vi "advent_5.vi"() -> ()   [LabVIEW 2021]
uses:
  <vilib>/Utility/file.llb/Read Delimited Spreadsheet (string).vi
panel:
  out "answer":i32
  out "Array 2":i32[][](array[numeric])
  out "Array":i32[][](array[numeric])
  out "ey":string[](array[string])
  out "ex":string[](array[string])
  out "e":string[](array[string])
  out "s":string[](array[string])
  out "sy":string[](array[string])
  out "sx":string[](array[string])
  out "all rows":string[][](array[string])
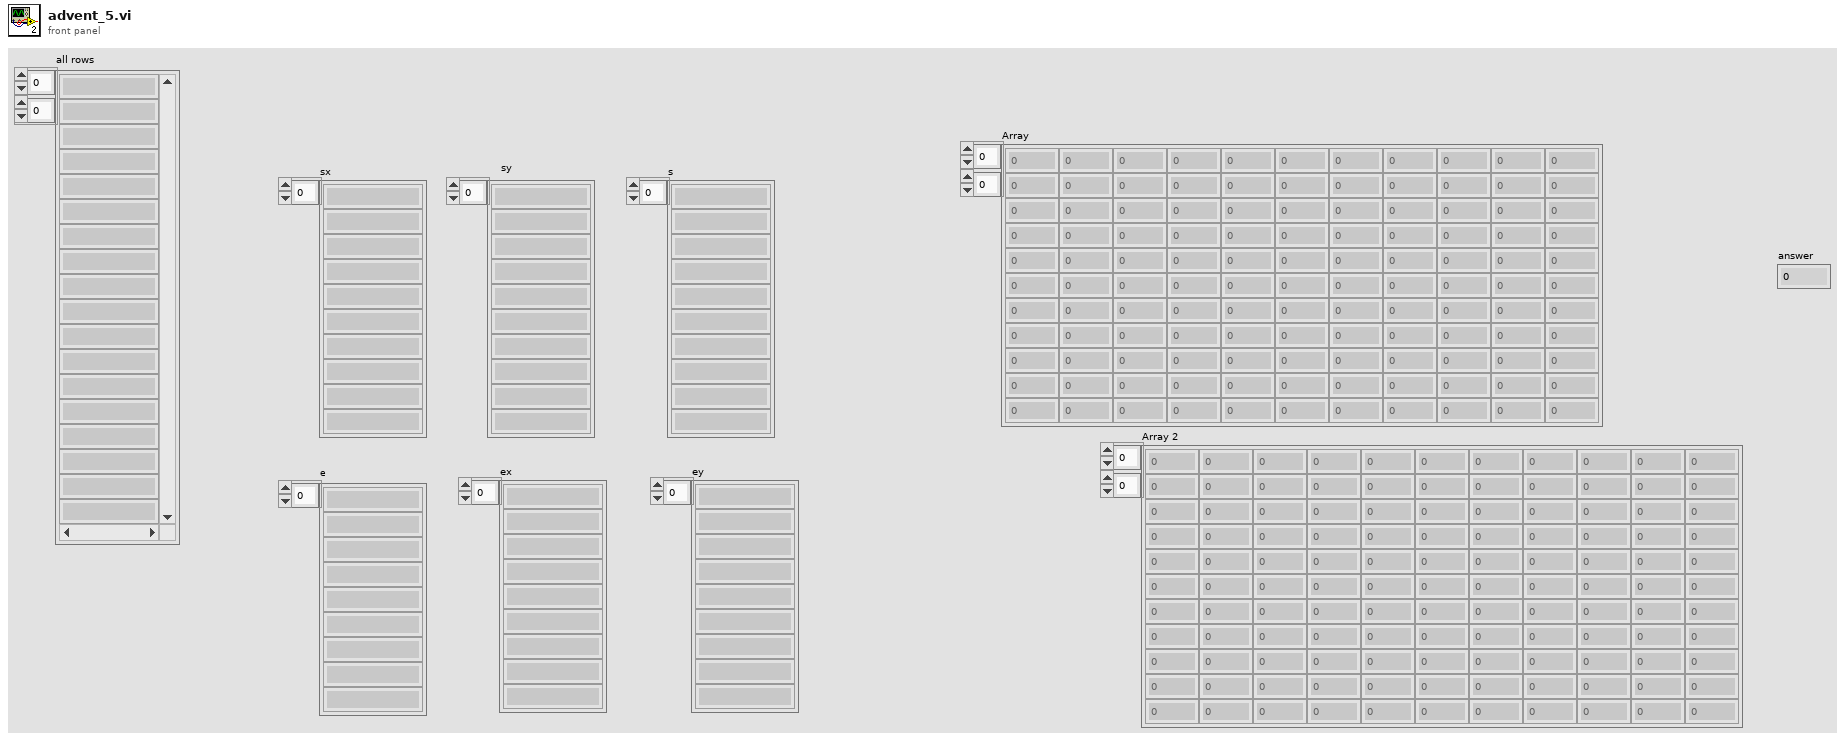
[diagram p1: front panel]
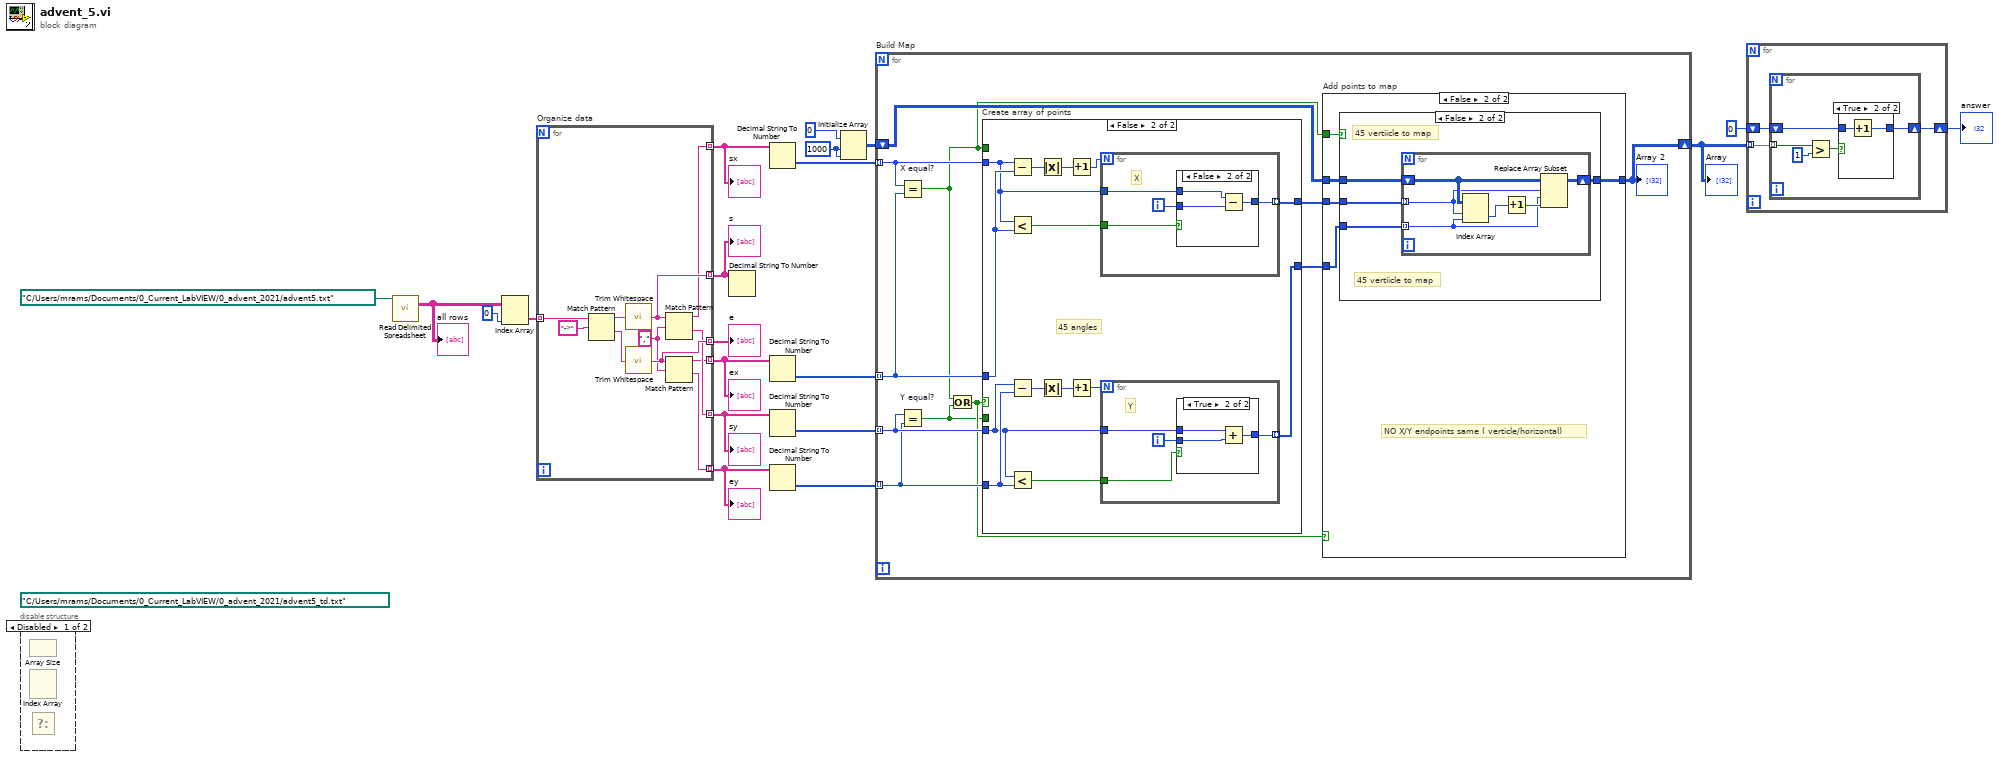
[diagram p0: block diagram]
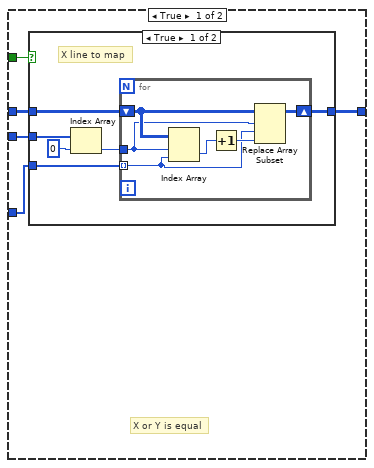
[diagram p3: hidden frame]
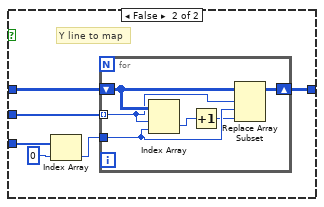
[diagram p4: hidden frame]
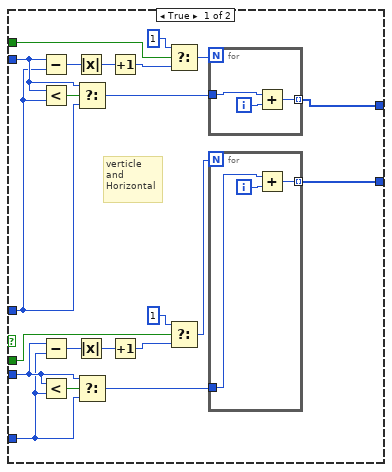
[diagram p6: hidden frame]
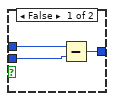
[diagram p7: hidden frame]
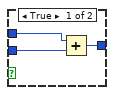
[diagram p8: hidden frame]
diagram:
  (unwired) path "C:/Users/mrams/Documents/0_Current_LabVIEW/0_advent_2021/advent5_td.txt" ("file path (dialog if empty)")
  w10 = 1000 ("dimension size")
  n1 = disable-structure shown="Disabled" {
    frame Disabled {
      n2 = Array Size() -> ()  [unwired: 1 in, 1 out]
      n3 = Index Array() -> ()  [unwired: 3 in, 1 out]
      n4 = Select() -> ()  [unwired: 3 in, 1 out]
    }
    frame Enabled {
    }
  }
  n5 = call-poly <vilib>:"Read Delimited Spreadsheet.vi"("file path (dialog if empty)"=path "C:/Users/mrams/Documents/0_Current_LabVIEW/0_advent_2021/advent5.txt") -> ("all rows"=w20:string[][])  [unwired: 9 in, 5 out]
  "all rows" <- w20
  n6 = Index Array(array=w20, index (col)=0 ("disabled index (col)")) -> (element=w18:string[])  [unwired: 1 in]
  n7 = for "Organize data" {
    tunnel: w18 -> [w31] mode=indexing
    tunnel: [w27] -> w14 mode=indexing
    tunnel: [w26] -> w17 mode=indexing
    tunnel: [w24] -> w16 mode=indexing
    tunnel: [w23] -> w15 mode=indexing
    tunnel: [w22] -> w13 mode=indexing
    tunnel: [w21] -> w12 mode=indexing
    w25 = "," ("regular expression")
    n8 = Match Pattern(string=w31, regular expression="->") -> (before substring=w29:string, after substring=w28:string)  [unwired: 1 in, 2 out]
    n9 = call <vilib>:"Trim Whitespace.vi"("string"=w29) -> ("trimmed string"=w27:string)  [unwired: 1 in]
    n10 = call <vilib>:"Trim Whitespace.vi"("string"=w28) -> ("trimmed string"=w26:string)  [unwired: 1 in]
    n11 = Match Pattern(string=w27, regular expression=w25) -> (before substring=w24:string, after substring=w23:string)  [unwired: 1 in, 2 out]
    n12 = Match Pattern(string=w26, regular expression=w25) -> (before substring=w22:string, after substring=w21:string)  [unwired: 1 in, 2 out]
  }
  "sx" <- w16
  "sy" <- w15
  "s" <- w14
  "e" <- w17
  "ex" <- w13
  "ey" <- w12
  n13 = Decimal String To Number(string=w14) -> ()  [unwired: 2 in, 2 out]
  n14 = Decimal String To Number(string=w16) -> (number=w9:i32[])  [unwired: 2 in, 1 out]
  n15 = Decimal String To Number(string=w13) -> (number=w8:i32[])  [unwired: 2 in, 1 out]
  n16 = Decimal String To Number(string=w15) -> (number=w7:i32[])  [unwired: 2 in, 1 out]
  n17 = Decimal String To Number(string=w12) -> (number=w6:i32[])  [unwired: 2 in, 1 out]
  n18 = Initialize Array(0, w10, w10) -> (w5:i32[][])
  n19 = for "Build Map" {
    tunnel: w9 -> [w42] mode=indexing
    tunnel: w8 -> [w41] mode=indexing
    tunnel: w7 -> [w40] mode=indexing
    tunnel: w6 -> [w39] mode=indexing
    shift-right: [w34] -> w4
    shift-left: w5 -> [w38]
    n20 = Equal? "X equal?"(x=w42, y=w41) -> (x = y?=w32:bool)
    n21 = Equal? "Y equal?"(x=w40, y=w39) -> (x = y?=w33:bool)
    n22 = Or(x=w32, y=w33) -> (x .or. y?=w36:bool)
    n23 = case "Create array of points" shown="False" w36 {
      tunnel: w42 -> [w108 w119]
      tunnel: w41 -> [w107 w129]
      tunnel: w40 -> [w103 w118]
      tunnel: w39 -> [w102 w128]
      tunnel: [w101 w127] -> w37
      tunnel: [w100 w126] -> w35
      tunnel: w33 -> [w99 _]
      tunnel: w32 -> [w95 _]
      frame True {
        # "verticle\nand\nHorizontal"
        n24 = Subtract(x=w108, y=w107) -> (x-y=w94:i32)
        n25 = Less?(x=w108, y=w107) -> (x < y?=w109:bool)
        n26 = Subtract(x=w103, y=w102) -> (x-y=w98:i32)
        n27 = Less?(x=w103, y=w102) -> (x < y?=w104:bool)
        n28 = Absolute Value(x=w94) -> (abs(x)=w91:i32)
        n29 = Absolute Value(x=w98) -> (abs(x)=w90:i32)
        n30 = Select(t=w108, s=w109, f=w107) -> (s? t:f=w106:i32)
        n31 = Select(t=w103, s=w104, f=w102) -> (s? t:f=w105:i32)
        n32 = Increment(x=w91) -> (x+1=w89:i32)
        n33 = Increment(x=w90) -> (x+1=w88:i32)
        n34 = Select(t=1, s=w95, f=w89) -> (s? t:f=w93:i32)
        n35 = Select(t=1, s=w99, f=w88) -> (s? t:f=w92:i32)
        n36 = for {
          N: w93 -> [_]
          tunnel: w106 -> [w115]
          tunnel: [w113] -> w100 mode=indexing
          i -> [w114]
          n37 = Add(x=w115, y=w114) -> (x+y=w113:i32)
        }
        n38 = for {
          N: w92 -> [_]
          tunnel: w105 -> [w112]
          tunnel: [w110] -> w101 mode=indexing
          i -> [w111]
          n39 = Add(x=w112, y=w111) -> (x+y=w110:i32)
        }
      }
      frame False {
        # "45 angles"
        n40 = Subtract(x=w119, y=w129) -> (x-y=w123:i32)
        n41 = Less?(x=w119, y=w129) -> (x < y?=w117:bool)
        n42 = Subtract(x=w118, y=w128) -> (x-y=w122:i32)
        n43 = Less?(x=w118, y=w128) -> (x < y?=w116:bool)
        n44 = Absolute Value(x=w123) -> (abs(x)=w125:i32)
        n45 = Absolute Value(x=w122) -> (abs(x)=w124:i32)
        n46 = Increment(x=w125) -> (x+1=w120:i32)
        n47 = Increment(x=w124) -> (x+1=w121:i32)
        n48 = for {
          N: w120 -> [_]
          tunnel: [w142] -> w126 mode=indexing
          tunnel: w119 -> [w140]
          tunnel: w117 -> [w141]
          i -> [w143]
          # "X"
          n49 = case shown="False" w141 {
            tunnel: w143 -> [w146 w149]
            tunnel: [w145 w148] -> w142
            tunnel: w140 -> [w144 w147]
            frame True {
              n50 = Add(x=w144, y=w146) -> (x+y=w145:i32)
            }
            frame False {
              n51 = Subtract(x=w147, y=w149) -> (x-y=w148:i32)
            }
          }
        }
        n52 = for {
          N: w121 -> [_]
          tunnel: [w132] -> w127 mode=indexing
          tunnel: w118 -> [w131]
          tunnel: w116 -> [w130]
          i -> [w133]
          # "Y"
          n53 = case shown="True" w130 {
            tunnel: w133 -> [w136 w139]
            tunnel: [w135 w138] -> w132
            tunnel: w131 -> [w134 w137]
            frame False {
              n54 = Subtract(x=w134, y=w136) -> (x-y=w135:i32)
            }
            frame True {
              n55 = Add(x=w137, y=w139) -> (x+y=w138:i32)
            }
          }
        }
      }
    }
    n56 = case "Add points to map" shown="False" w36 {
      tunnel: w32 -> [w47 w76]
      tunnel: w38 -> [w46 w75]
      tunnel: w37 -> [w45 w74]
      tunnel: w35 -> [w44 w73]
      tunnel: [w43 w72] -> w34
      frame True {
        # "X or Y is equal"
        n57 = case shown="True" w47 {
          tunnel: w46 -> [w52 w61]
          tunnel: w45 -> [w48 w64]
          tunnel: w44 -> [w50 w65]
          tunnel: [w51 w60] -> w43
          frame True {
            # "X line to map"
            n58 = Index Array(array=w50, index=0) -> (element=w49:i32)
            n59 = for {
              shift-right: [w56] -> w51
              shift-left: w52 -> [w59]
              tunnel: w49 -> [w54]
              tunnel: w48 -> [w55] mode=indexing
              n60 = Index Array(array=w59, index (row)=w54, index (col)=w55) -> (element=w58:i32)
              n61 = Increment(x=w58) -> (x+1=w57:i32)
              n62 = Replace Array Subset(array=w59, new element=w57, index (row)=w54, index (col)=w55) -> (w56:i32[][])
            }
          }
          frame False {
            # "Y line to map"
            n63 = Index Array(array=w64, index=0) -> (element=w62:i32)
            n64 = for {
              tunnel: w65 -> [w69] mode=indexing
              tunnel: w62 -> [w68]
              shift-right: [w66] -> w60
              shift-left: w61 -> [w71]
              n65 = Index Array(array=w71, index (row)=w69, index (col)=w68) -> (element=w70:i32)
              n66 = Increment(x=w70) -> (x+1=w67:i32)
              n67 = Replace Array Subset(array=w71, new element=w67, index (row)=w69, index (col)=w68) -> (w66:i32[][])
            }
          }
        }
      }
      frame False {
        # "NO X/Y endpoints same ( verticle/horizontal)"
        n68 = case shown="False" w76 {
          tunnel: w75 -> [w77 w80]
          tunnel: w74 -> [_ w78]
          tunnel: w73 -> [_ w81]
          tunnel: [w77 w79] -> w72
          frame True {
            # "never fires"
          }
          frame False {
            # "45 vertiicle to map"
            # "45 vertiicle to map"
            n69 = for {
              tunnel: w81 -> [w85] mode=indexing
              shift-right: [w83] -> w79
              shift-left: w80 -> [w87]
              tunnel: w78 -> [w82] mode=indexing
              n70 = Index Array(array=w87, index (row)=w85, index (col)=w82) -> (element=w86:i32)
              n71 = Increment(x=w86) -> (x+1=w84:i32)
              n72 = Replace Array Subset(array=w87, new element=w84, index (row)=w85, index (col)=w82) -> (w83:i32[][])
            }
          }
        }
      }
    }
    "Array 2" <- w34
  }
  "Array" <- w4
  n73 = for {
    tunnel: w4 -> [w152] mode=indexing
    shift-right: [w150] -> w2
    shift-left: 0 -> [w151]
    n74 = for {
      tunnel: w152 -> [w157] mode=indexing
      shift-right: [w153] -> w150
      shift-left: w151 -> [w154]
      n75 = Greater?(x=w157, y=1) -> (0:w155:bool)
      n76 = case shown="True" w155 {
        tunnel: w154 -> [w158 w160]
        tunnel: [w158 w159] -> w153
        frame False {
        }
        frame True {
          n77 = Increment(x=w160) -> (x+1=w159:i32)
        }
      }
    }
  }
  "answer" <- w2
